vi "BooleanArrayToStr(cast).vi"(1 "布尔数组":bool[](array[boolean])) -> (0 "字符串":string)   [LabVIEW 2012]
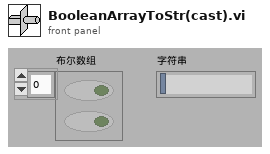
[diagram p1: front panel]
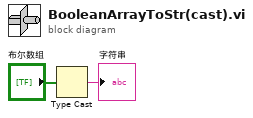
[diagram p0: block diagram]
diagram:
  n1 = Type Cast(x="布尔数组") -> (*(type *) &x=→"字符串":string)  [unwired: 1 in]
